vi "ArrayComplexCsgToImage.vi"(8 "error in":errorcluster, 10 "Pixel":csg[][](array[numeric]), 11 "Image Reference In":T1) -> (0 "error out":errorcluster, 3 "Image Reference Out":T1)   [LabVIEW 2020, in "OpenLvVision_Image.lvlib" / "DataAccess.lvlib"]
doc: "Replaces the image's data with the provided array (Copy)"
uses:
  DataAccess.lvlib
  Management/TypeDef/Image.ctl
  Management/Management.lvlib
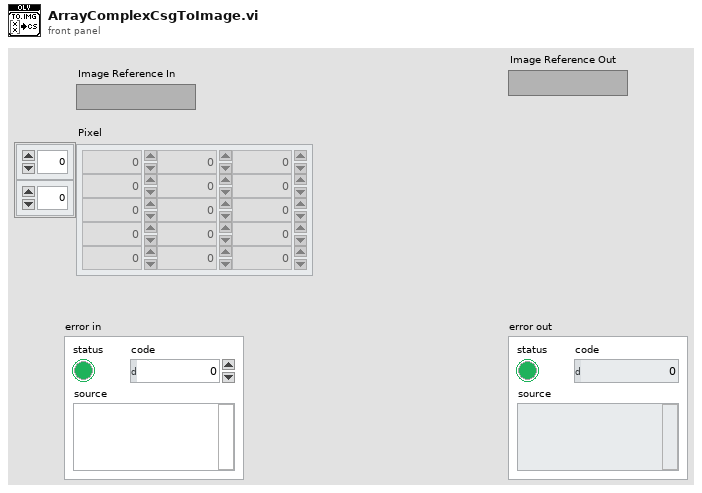
[diagram p1: front panel]
types:
  T1 = typedef "OpenLvVision_Image.lvlib/Management.lvlib/Image.ctl" = refnum<image>
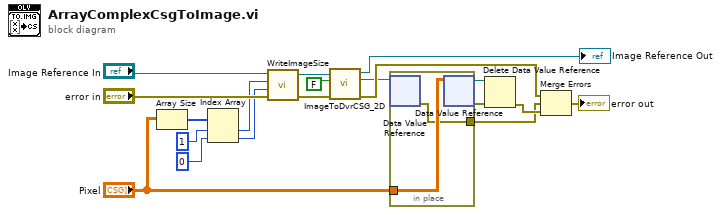
[diagram p0: block diagram]
diagram:
  n1 = Array Size(array="Pixel") -> (size(s)=w14:i32[])
  n2 = Index Array(array=w14, index #1=1, index #2=0) -> (element #1=w13:i32, element #2=w12:i32)
  n3 = call "WriteImageSize.vi"("error in"="error in", "Height"=w12, "Width"=w13, "Image Reference In"="Image Reference In") -> ("error out"=w15:errorcluster, "Image Reference Out"=w16:T1)  [unwired: 6 in]
  n4 = call "ImageToDvrCSG_2D.vi"("error in"=w15, "Include Border"=FALSE, "Image Reference In"=w16) -> ("error out"=w6:errorcluster, "EDVR 2D CSG"=w5:refnum<data-value>, "Image Reference Out"=→"Image Reference Out":T1)  [unwired: 5 in, 1 out]
  n5 = in-place {
    in-place-border: "Pixel" -> [w21]
    in-place-border: [w20] -> w3
    n6 = in-place-dvr #1(w5) -> (w20:errorcluster)  [unwired: 1 out]
    n7 = in-place-dvr #1(w21) -> (w9:refnum<data-value>, w10:errorcluster)
  }
  n8 = Delete Data Value Reference(data value reference=w9, error in=w10) -> (error out=w4:errorcluster)  [unwired: 1 out]
  n9 = Merge Errors(w6, w3, w4) -> (→"error out":errorcluster)
